vi "setChannelDefaultValues.vi"(8 "error in (no error)":errorcluster, 9 "calibratedValues":dbl[](array[numeric]) format="%.8g", 10 "channel_addresses":string[](array[string]), 11 "AnalogOutput in":refnum<class "AnalogOutput.lvclass">) -> (0 "error out":errorcluster, 3 "AnalogOutput out":refnum<class "AnalogOutput.lvclass">)   [LabVIEW 2009, in "Hardware.lvlib" / "Channels.lvlib" / "AnalogOutput.lvclass"]
uses:
  AnalogOutput.lvclass
  AnalogOutput.lvclass/AnalogOutput.ctl
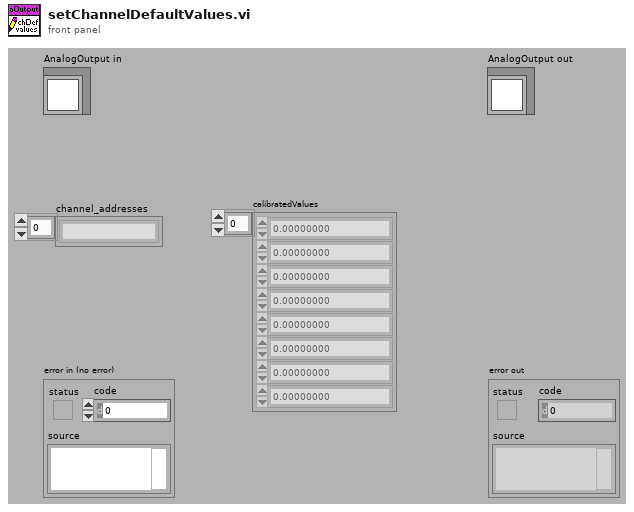
[diagram p1: front panel]
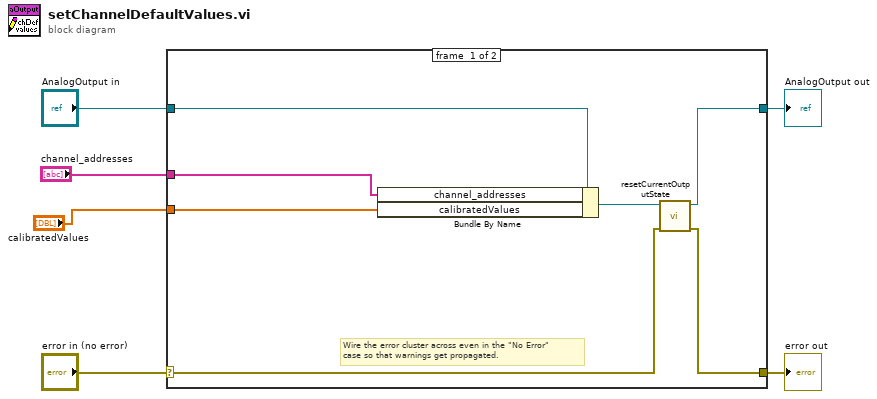
[diagram p0: block diagram]
diagram:
  n1 = case shown="No Error" "error in (no error)" {
    selector: "error in (no error)" -> [w8 w15]
    tunnel: [w7 w15] -> w5
    tunnel: [w9 w14] -> w3
    tunnel: "AnalogOutput in" -> [w13 w14]
    tunnel: "channel_addresses" -> [w12 _]
    tunnel: "calibratedValues" -> [w11 _]
    frame #0 {
      # "Wire the error cluster across even in the \"No Error\"\ncase so that warnings get propagated."
      n2 = Bundle By Name(cluster=w13, "channel_addresses"=w12, "calibratedValues"=w11) -> (w10:refnum<class "AnalogOutput.lvclass">)
      n3 = call "resetCurrentOutputState.vi"("error in (no error)"=w8, "AnalogOutput in"=w10) -> ("error out"=w7:errorcluster, "AnalogOutput out"=w9:refnum<class "AnalogOutput.lvclass">)  [unwired: 8 in]
    }
    frame #1 {
    }
  }
  "error out" <- w5
  "AnalogOutput out" <- w3
